vi "Pockels-Modify intensity.vi"(9 "Pockels control value (V)":dbl) -> (0 "error out":errorcluster, 1 "Modified data":dbl[](array[numeric]))   [LabVIEW 2013]
uses:
  Typedefs/Functional Global Default States.ctl
  <vilib>/DAQmx/write.llb/DAQmx Write (Analog 1D DBL 1Chan NSamp).vi
  Program Files (x86)/National Instruments/LabVIEW 2013/user.lib/_OpenG.lib/array/array.llb/Search 1D Array (DBL)__ogtk.vi
  Triggers/Globals/gl_Triggering globals.vi
  <vilib>/DAQmx/miscellaneous.llb/DAQmx Fill In Error Info.vi
panel:
  out "Waveform Graph":dbl[](graph)
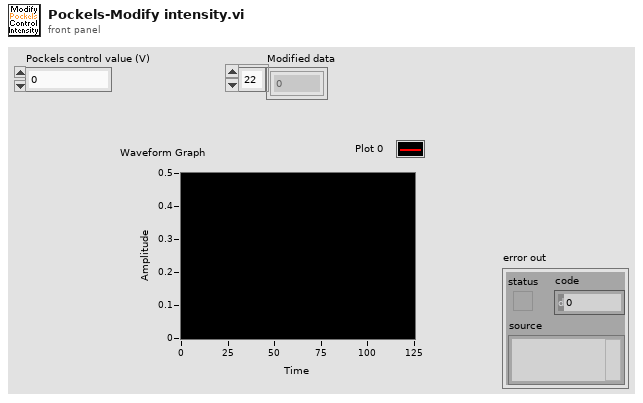
[diagram p1: front panel]
types:
  T1 = typedef "Functional Global Default States.ctl" = enum16{"Read", "Write", "Clear"}
  T2 = typedef "Triggered tasks cluster.ctl" = cluster{"DO task-Encoder trigger":refnum<k21>, "AO Task-Pockels modulation":refnum<k21>, "Counter Clock Task":refnum<k21>}
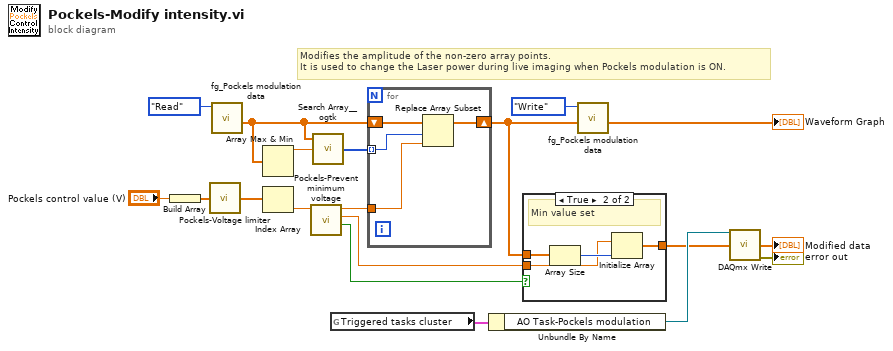
[diagram p0: block diagram]
diagram:
  # "Modifies the amplitude of the non-zero array points.\nIt is used to change the Laser power during live imaging when Pockels modulation is ON."
  n1 = Build Array("Pockels control value (V)") -> (w13:dbl[])
  n2 = call "Pockels-Voltage limiter.vi"("Pockels AO data in"=w13) -> ("Pockels AO data out"=w12:dbl[])
  n3 = call "fg_Pockels modulation data.vi"("Function"=Functional_Global_Default_States."Read") -> ("Pockels modulation data out"=w1:dbl[])  [unwired: 10 in]
  n4 = Array Max & Min(array=w1) -> (max value=w17:dbl)  [unwired: 3 out]
  n5 = Index Array(array=w12) -> (element=w10:dbl)  [unwired: 1 in]
  n6 = call "Pockels-Prevent minimum voltage.vi"("Pockels Value"=w10) -> ("Minimum voltage attempt"=w8:bool, "Pockels voltage min"=w7:dbl, "Pockels Value (minimum prevented)"=w9:dbl)  [unwired: 8 in]
  n7 = call-poly "Search Array__ogtk.vi"("Array"=w1, "Element Data"=w17) -> ("Indices of Elements"=w18:i32[])  [unwired: 7 in]
  n8 = global read "gl_Triggering globals.vi" "Triggered tasks cluster"() -> (w16:T2)
  n9 = for {
    tunnel: w18 -> [w20] mode=indexing
    shift-right: [w19] -> w4
    shift-left: w1 -> [w22]
    tunnel: w9 -> [w21]
    n10 = Replace Array Subset(array=w22, new element=w21, index=w20) -> (w19:dbl[])
  }
  n11 = Unbundle By Name(w16) -> ("AO Task-Pockels modulation"=w14:refnum<k21>)
  n12 = case shown="True" w8 {
    tunnel: w4 -> [w23 w27]
    tunnel: w7 -> [_ w25]
    tunnel: [w23 w24] -> w6
    frame False {
    }
    frame True {
      # "Min value set"
      n13 = Array Size(array=w27) -> (size(s)=w26:i32)
      n14 = Initialize Array(w25, w26) -> (w24:dbl[])
    }
  }
  "Modified data" <- w6
  n15 = call "fg_Pockels modulation data.vi"("Pockels modulation data in"=w4, "Function"=Functional_Global_Default_States."Write") -> ("Pockels modulation data out"=→"Waveform Graph":dbl[])  [unwired: 9 in]
  n16 = call-poly <vilib>:"DAQmx Write.vi"("task/channels in"=w14, "data"=w6) -> ("error out"=→"error out":errorcluster)  [unwired: 11 in, 2 out]
